vi "Read_Register.vi"(8 "error in (no error)":errorcluster, 11 "Serial Config":T1={"Baud"=9600, "Flow Ctl"=0, "Parity"=0, "Address"=1, "VISA resource name"=""} {"Parity" items=["None", "Odd", "Even"]; "Flow Ctl" items=["None"]; "Baud" items=["4800"=4800, "9600"=9600, "19200"=19200, "38400"=38400]}) -> (0 "error out":errorcluster, 3 "Serial Config out":T1={"Baud"=9600, "Flow Ctl"=0, "Parity"=0, "Address"=0, "VISA resource name"=""} {"Parity" items=["None", "Odd", "Even"]; "Flow Ctl" items=["None"]; "Baud" items=["4800"=4800, "9600"=9600, "19200"=19200, "38400"=38400]})   [LabVIEW 2014, in "Omega CN9600 series.lvclass"]
uses:
  Omega CN9600 series.lvclass
  Serial_Config_Omega.ctl
panel:
  out "Value":u16
  in  "Address":u16 format="%x"
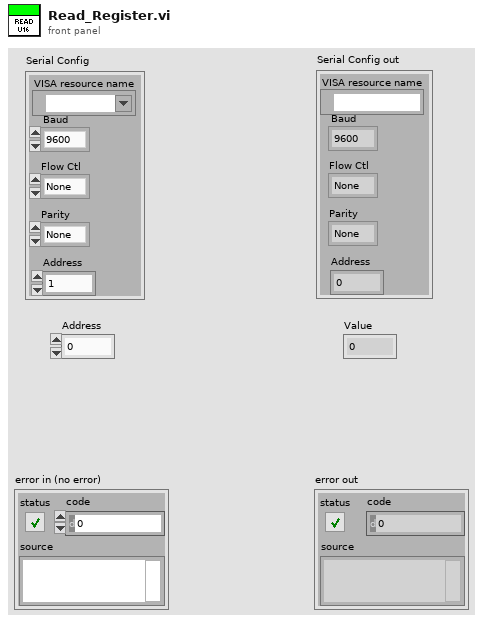
[diagram p1: front panel]
types:
  T1 = typedef "Omega CN9600 series.lvclass/Serial_Config_Omega.ctl" = cluster{"Baud":u32, "Flow Ctl":u16, "Parity":u16, "Address":u8, "VISA resource name":refnum<visa-resource-name>}
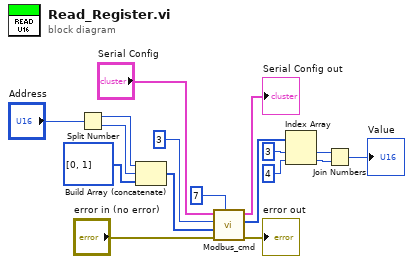
[diagram p0: block diagram]
diagram:
  n1 = Split Number(x="Address") -> (hi(x)=w11:u8, lo(x)=w9:u8)
  n2 = Build Array (concatenate)(w11, w9, u8[] [0, 1] ("Data")) -> (w8:u8[])
  n3 = call "Modbus_cmd.vi"("Bytes to read"=u32 7, "error in (no error)"="error in (no error)", "Data"=w8, "Function"=u8 3, "Serial Config"="Serial Config") -> ("error out"=→"error out":errorcluster, "Response"=w6:u8[], "Serial Config out"=→"Serial Config out":T1)  [unwired: 3 in, 1 out]
  n4 = Index Array(array=w6, index #1=3 ("index"), index #2=4 ("index")) -> (element #1=w3:u8, element #2=w2:u8)
  n5 = Join Numbers(hi=w3, lo=w2) -> ((hi.lo)=→"Value":u16)
